vi "HOST_feedback+datatrig_AAoptAOD_9-20-23.vi"() -> ()   [LabVIEW 2020]
uses:
  <vilib>/rvi/interface/nirviMethod/nirviMethod.xnode
  <vilib>/rvi/errors/niLvFpgaMergeErrorWithErrorCode.vi
  <instrlib>/_niInstr/Streaming/v1/Host/niInstr Streaming v1 Host.lvlib
  <vilib>/rvi/interface/nirviReadWriteControl/nirviReadWriteControl.xnode
  <vilib>/rvi/interface/nirviCloseFPGA/nirviCloseFPGA.xnode
  <vilib>/rvi/interface/nirviOpenFPGA/nirviOpenFPGA.xnode
  <vilib>/rvi/interface/Simulation/niFpgaSimulationCallBeginRW.vi
  <vilib>/rvi/errors/niLvFpgaAdjustHostInterfaceError.vi
  NiFpgaLv.dll
  <vilib>/Utility/error.llb/Error Cluster From Error Code.vi
  <vilib>/Utility/file.llb/Write Delimited Spreadsheet (string).vi
  <instrlib>/_niInstr/Streaming/v1/Host/Public/Start Finite Stream.vi
  <instrlib>/_niInstr/Streaming/v1/Host/Public/Wait for Stream.vi
  <vilib>/FPGAPlugInAG/Dynamic/niLvFpga_ConfigureFifo_Dynamic.vi
  <vilib>/FPGAPlugInAG/Dynamic/niLvFpga_StartFifo_Dynamic.vi
  <vilib>/measure/NI_MAPro.lvlib
  <vilib>/measure/maspectr.llb/FFT Power Spectrum and PSD for N Chan.vi
  <instrlib>/_niInstr/Streaming/v1/Host/Public/Start Continuous Stream.vi
  <vilib>/FPGAPlugInAG/Dynamic/niLvFpga_ReadFifo_Dynamic.vi
  <vilib>/FPGAPlugInAG/Dynamic/niLvFpga_WriteFifo_Dynamic.vi
  <vilib>/FPGAPlugInAG/Dynamic/niLvFpga_Close_Dynamic.vi
  FPGA Bitfiles/rfsignalsimplifi_FPGATarget_feedbackarray+da_Q0z18vTqQOY.lvbitx
  <vilib>/FPGAPlugInAG/PXIe-7972R/niLvFpga_Open_PXIe-7972R.vi
  <vilib>/rvi/interface/common/dynamic/niFpgaDynamicAddResources.vi
  <vilib>/userdefined/Silver/nirio_resource_slv.ctl
  Controls/Clock Select.ctl
  PID/Typedef/niFpgaPID_PIDGains_FXP.ctl
  PID/Typedef/niFpgaPID_SetpointWeightings_FXP.ctl
  PID/Typedef/niFpgaPID_OutputRange_FXP.ctl
  PID/Typedef/niFpgaPID_PIDActions_FXP.ctl
panel:
  out "Boolean":bool=TRUE
  out "Stream PSD":cluster{"f0":dbl, "df":dbl, "magnitude":dbl[]}[](graph)
  out "X DC Offset Check":i16[](array[numeric])
  in  "Number of files":u16=1
  in  "RF Power normalize":bool=TRUE
  in  "Save data":bool
  in  "File base name":string="Z_3mbar_i"
  in  "Save Path Directory":path=path "D:/Lab Data/test"
  out "SUM PSD":cluster{"f0":dbl, "df":dbl, "magnitude":dbl[]}[](graph)
  out "SUM":waveform(dbl)[](graph)=[{"t0"=timestamp(0 s since 1904-01-01), "dt"=0.0002, "Y"=array[1000 elements]}, {"t0"=timestamp(0 s since 1904-01-01), "dt"=0.0002, "Y"=array[1000 elements]}, {"t0"=timestamp(0 s since 1904-01-01), "dt"=0.0002, "Y"=array[1000 elements]}, {"t0"=timestamp(0 s since 1904-01-01), "dt"=0.0002, "Y"=array[1000 elements]}]
  out "Y PSD":cluster{"f0":dbl, "df":dbl, "magnitude":dbl[]}[](graph)
  out "Y":waveform(dbl)[](graph)=[{"t0"=timestamp(0 s since 1904-01-01), "dt"=0.0002, "Y"=array[1000 elements]}, {"t0"=timestamp(0 s since 1904-01-01), "dt"=0.0002, "Y"=array[1000 elements]}, {"t0"=timestamp(0 s since 1904-01-01), "dt"=0.0002, "Y"=array[1000 elements]}, {"t0"=timestamp(0 s since 1904-01-01), "dt"=0.0002, "Y"=array[1000 elements]}]
  out "X PSD":cluster{"f0":dbl, "df":dbl, "magnitude":dbl[]}[](graph)
  out "X":waveform(dbl)[](graph)=[{"t0"=timestamp(0 s since 1904-01-01), "dt"=0.0002, "Y"=array[1000 elements]}, {"t0"=timestamp(0 s since 1904-01-01), "dt"=0.0002, "Y"=array[1000 elements]}, {"t0"=timestamp(0 s since 1904-01-01), "dt"=0.0002, "Y"=array[1000 elements]}, {"t0"=timestamp(0 s since 1904-01-01), "dt"=0.0002, "Y"=array[1000 elements]}]
  in  "Set Point Initialization":bool
  in  "Feedback scaling y":fxp<+,25,4>
  in  "Y Gains":T1[](array[typedef])
  in  "X Gains":T1[](array[typedef])
  in  "Data transfer method":bool
  in  "Downsample":u16=1
  in  "Signal Delay (us)":u16=5
  out "actions":T2
  out "error":fxp<+/-,18,11>
  out "output":fxp<+/-,20,12>
  out "error 2":fxp<+/-,18,11>
  out "error 3":fxp<+/-,18,11>
  out "output 3":fxp<+/-,20,12>
  out "actions 3":T2
  out "output 2":fxp<+/-,20,12>
  out "actions 2":T2
  in  "Z Gains":T1[](array[typedef])
  in  "setpoint weighting 3":T3={"proportional weighting (1)"=1.0, "derivative weighting (0)"=0.0}
  in  "output range 3":T4={"output high (Inf)"=2000.0, "output low (-Inf)"=-2000.0}
  in  "Z reset? (F)":bool
  in  "setpoint weighting 2":T3={"proportional weighting (1)"=1.0, "derivative weighting (0)"=0.0}
  in  "output range 2":T4={"output high (Inf)"=2000.0, "output low (-Inf)"=-2000.0}
  in  "Y reset? (F)":bool
  in  "Feedback scaling z":fxp<+,32,4>
  in  "Feedback scaling x":fxp<+,25,4>
  in  "Apply feedback":bool
  in  "Data Trigger Level (V)":dbl
  in  "Record Size":u32=1024
  out "AI":waveform(dbl)[](graph)
  in  "Data Trigger When":enum8{"Trigger Above", "Trigger Below"}(ring)
  in  "Trigger Type":enum8{"Immediate", "Data Trigger", "TRIG input"}(ring)
  in  "Direction switch":bool
  in  "Step gain values":dbl
  in  "?":bool
  in  "% of max CH 1":dbl=85.0
  in  "% of max CH 0":dbl=90.0
  in  "setpoint weighting":T3={"proportional weighting (1)"=1.0, "derivative weighting (0)"=0.0}
  in  "output range":T4={"output high (Inf)"=2000.0, "output low (-Inf)"=-2000.0}
  in  "X reset? (F)":bool
  in  "write time ch0":bool
  in  "Record time for power sweep CH0":bool
  in  "Record time for power sweep CH1":bool
  in  "write time ch1":bool
  in  "save path for power calibration (dialog if empty)":path
  out "time check":u16=16
  in  "Cycles per step":u16=30
  in  "Gain Scan Endpoint (CH1)":dbl[](array[numeric])=[100.0, 100.0, 100.0, 100.0, 100.0, 100.0, 100.0, 100.0, 100.0, 100.0, 100.0, 100.0, 100.0, 100.0, 100.0, 100.0, 100.0, 100.0, 100.0, 100.0, 100.0, 100.0, 100.0, 100.0, 100.0, 100.0, 100.0, 100.0, 100.0, 100.0, 100.0, 100.0, 100.0, 100.0, 100.0, 100.0]
  in  "Gain Scan Endpoint (CH0)":dbl[](array[numeric])=[100.0, 100.0, 100.0, 100.0, 100.0, 100.0, 100.0, 100.0, 100.0, 100.0, 100.0, 100.0, 100.0, 100.0, 100.0, 100.0, 100.0, 100.0, 100.0, 100.0, 100.0, 100.0, 100.0, 100.0, 100.0, 100.0, 100.0, 100.0, 100.0, 100.0, 100.0, 100.0, 100.0, 100.0, 100.0, 100.0]
  in  "Scan End Setpoint (CH1)":dbl[](array[numeric])=[23.0, 24.0, 25.0, 26.0, 27.0, 28.0, 23.0, 24.0, 25.0, 26.0, 27.0, 28.0, 23.0, 24.0, 25.0, 26.0, 27.0, 28.0, 23.0, 24.0, 25.0, 26.0, 27.0, 28.0, 23.0, 24.0, 25.0, 26.0, 27.0, 28.0, 23.0, 24.0, 25.0, 26.0, 27.0, 28.0] format="%#_10f"
  in  "Scan CH1":bool
  in  "Scan CH0":bool
  in  "Fq Scan Endpoint (CH0)":dbl[](array[numeric])=[23.0, 23.0, 23.0, 23.0, 23.0, 23.0, 24.0, 24.0, 24.0, 24.0, 24.0, 24.0, 25.0, 25.0, 25.0, 25.0, 25.0, 25.0, 26.0, 26.0, 26.0, 26.0, 26.0, 26.0, 27.0, 27.0, 27.0, 27.0, 27.0, 27.0, 28.0, 28.0, 28.0, 28.0, 28.0, 28.0] format="%#_10f"
  in  "Gain Scan Step Size % (CH1)":dbl=1.0
  in  "Gain Scan Step Size % (CH0)":dbl=1.0
  in  "Fq Scan Step Size MHz (CH1)":dbl=0.1
  in  "Fq Scan Step Size MHz (CH0)":dbl=0.1
  in  "Input pass through\nmode":enum16{"Wire", "Accum-edge"}(ring)=enum."Accum-edge"
  in  "# of beams":u8=36
  in  "Wave Reader CH 1 (MHz)":dbl[](array[numeric])=[23.0, 24.0, 25.0, 26.0, 27.0, 28.0, 23.0, 24.0, 25.0, 26.0, 27.0, 28.0, 23.0, 24.0, 25.0, 26.0, 27.0, 28.0, 23.0, 24.0, 25.0, 26.0, 27.0, 28.0, 23.0, 24.0, 25.0, 26.0, 27.0, 28.0, 23.0, 24.0, 25.0, 26.0, 27.0, 28.0] format="%#_15f"
  in  "Gain CH 1 (%)":dbl[](array[numeric])=[100.0, 100.0, 100.0, 100.0, 100.0, 100.0, 100.0, 100.0, 100.0, 100.0, 100.0, 100.0, 100.0, 100.0, 100.0, 100.0, 100.0, 100.0, 100.0, 100.0, 100.0, 100.0, 100.0, 100.0, 100.0, 100.0, 100.0, 100.0, 100.0, 100.0, 100.0, 100.0, 100.0, 100.0, 100.0, 100.0]
  in  "Remove transition edges":u16=5
  in  "Time per beam in us":u16=20
  in  "stop":bool
  in  "Gain CH 0 (%)":dbl[](array[numeric])=[100.0, 100.0, 100.0, 100.0, 100.0, 100.0, 100.0, 100.0, 100.0, 100.0, 100.0, 100.0, 100.0, 100.0, 100.0, 100.0, 100.0, 100.0, 100.0, 100.0, 100.0, 100.0, 100.0, 100.0, 100.0, 100.0, 100.0, 100.0, 100.0, 100.0, 100.0, 100.0, 100.0, 100.0, 100.0, 100.0]
  in  "Wave Reader CH 0 (MHz)":dbl[](array[numeric])=[23.0, 23.0, 23.0, 23.0, 23.0, 23.0, 24.0, 24.0, 24.0, 24.0, 24.0, 24.0, 25.0, 25.0, 25.0, 25.0, 25.0, 25.0, 26.0, 26.0, 26.0, 26.0, 26.0, 26.0, 27.0, 27.0, 27.0, 27.0, 27.0, 27.0, 28.0, 28.0, 28.0, 28.0, 28.0, 28.0] format="%#_13f"
  in  "Magnitude Initialization Vpp":dbl[](array[numeric])=[1.0, 1.0] format="%0.2p"
  in  "Frequencies (Hz)":dbl[](array[numeric])=[10000.0, 10000.0] format="%5.0p"
  in  "Signal Type":T5(ring)
  in  "Sampling Info":cluster{"Fs":dbl, "#s":dbl}={"Fs"=163840000.0, "#s"=32768.0} {"Fs" format="%#_5p"}
  out "Error Out":errorcluster
  in  "Update Waveform":bool
  in  "Clock Select":T6 items=["Internal Clock", "Internal Clock w/ Ref via CLK/REF IN", "Internal Clock w/ Ref via Sync Clock", "External Clock via CLK/REF IN"]
  in  "Rate of External Sample Clock (MHz)":u16=100 min=60 max=100 step=1
  in  "RIO Resource":T7="RIO0"
  # "For collecting the time and frequency when doing calibration"
  # "General Feedback Settings"
  # "Time cycle loop processing"
  # "up to 65535"
  # "Waveform Initialization"
  # "Controls the Output of the FPGA\nEach row corresponds to one beam created by the AOD\nCH 0 is Output 0 on the FPGA card and controls the () direction on the AOD; CH 1 is Output 1 on the FPGA card and controls the () direction on the AOD\n\nThe  set frequency is the output of the FPGA, this is then mixed with a 50MHz LO to be in the AOD's bandwidth of 75 +- 15MHz\n\nThe gain is the percentage of the 1Vpp initialized voltage to output. It is in percentage and goes from 0 - 100\n\nIt will play the first n rows of tones, \nwhere n is the \"# of beams\" value."
  # "DO NOT CHANGE"
  # "These allow you to smoothly ramp between frequencies or gain settings for each individual beam.\nThe channels scan independently, but it will simultaneously ramp every fq/gain in the channel to their desired point.\nThey should update to match the main control setting when scanning is not enabled."
  # "X Feedback"
  # "Do not change these values while waiting for scan"
  # "Main control for the tones played on FPGA analog out 0\nSets the base, static frequency to play"
  # "Main control for the tones played on FPGA analog out 1\nSets the base, static frequency to play"
  # "Don't change"
  # "Ch 0 Output Waveforms"
  # "Ch 1 Output Waveforms"
  # "Y Feedback"
  # "Ch0"
  # "Ch1"
  # "Makes sure the RF power into the\nAOD is flattened to 1.7W across the\nbandwidth\nDO NOT TURN OFF UNLESS YOU\nARE CALIBRATING POWERS!\nWILL BREAK THE AOD!"
  # "Z Feedback"
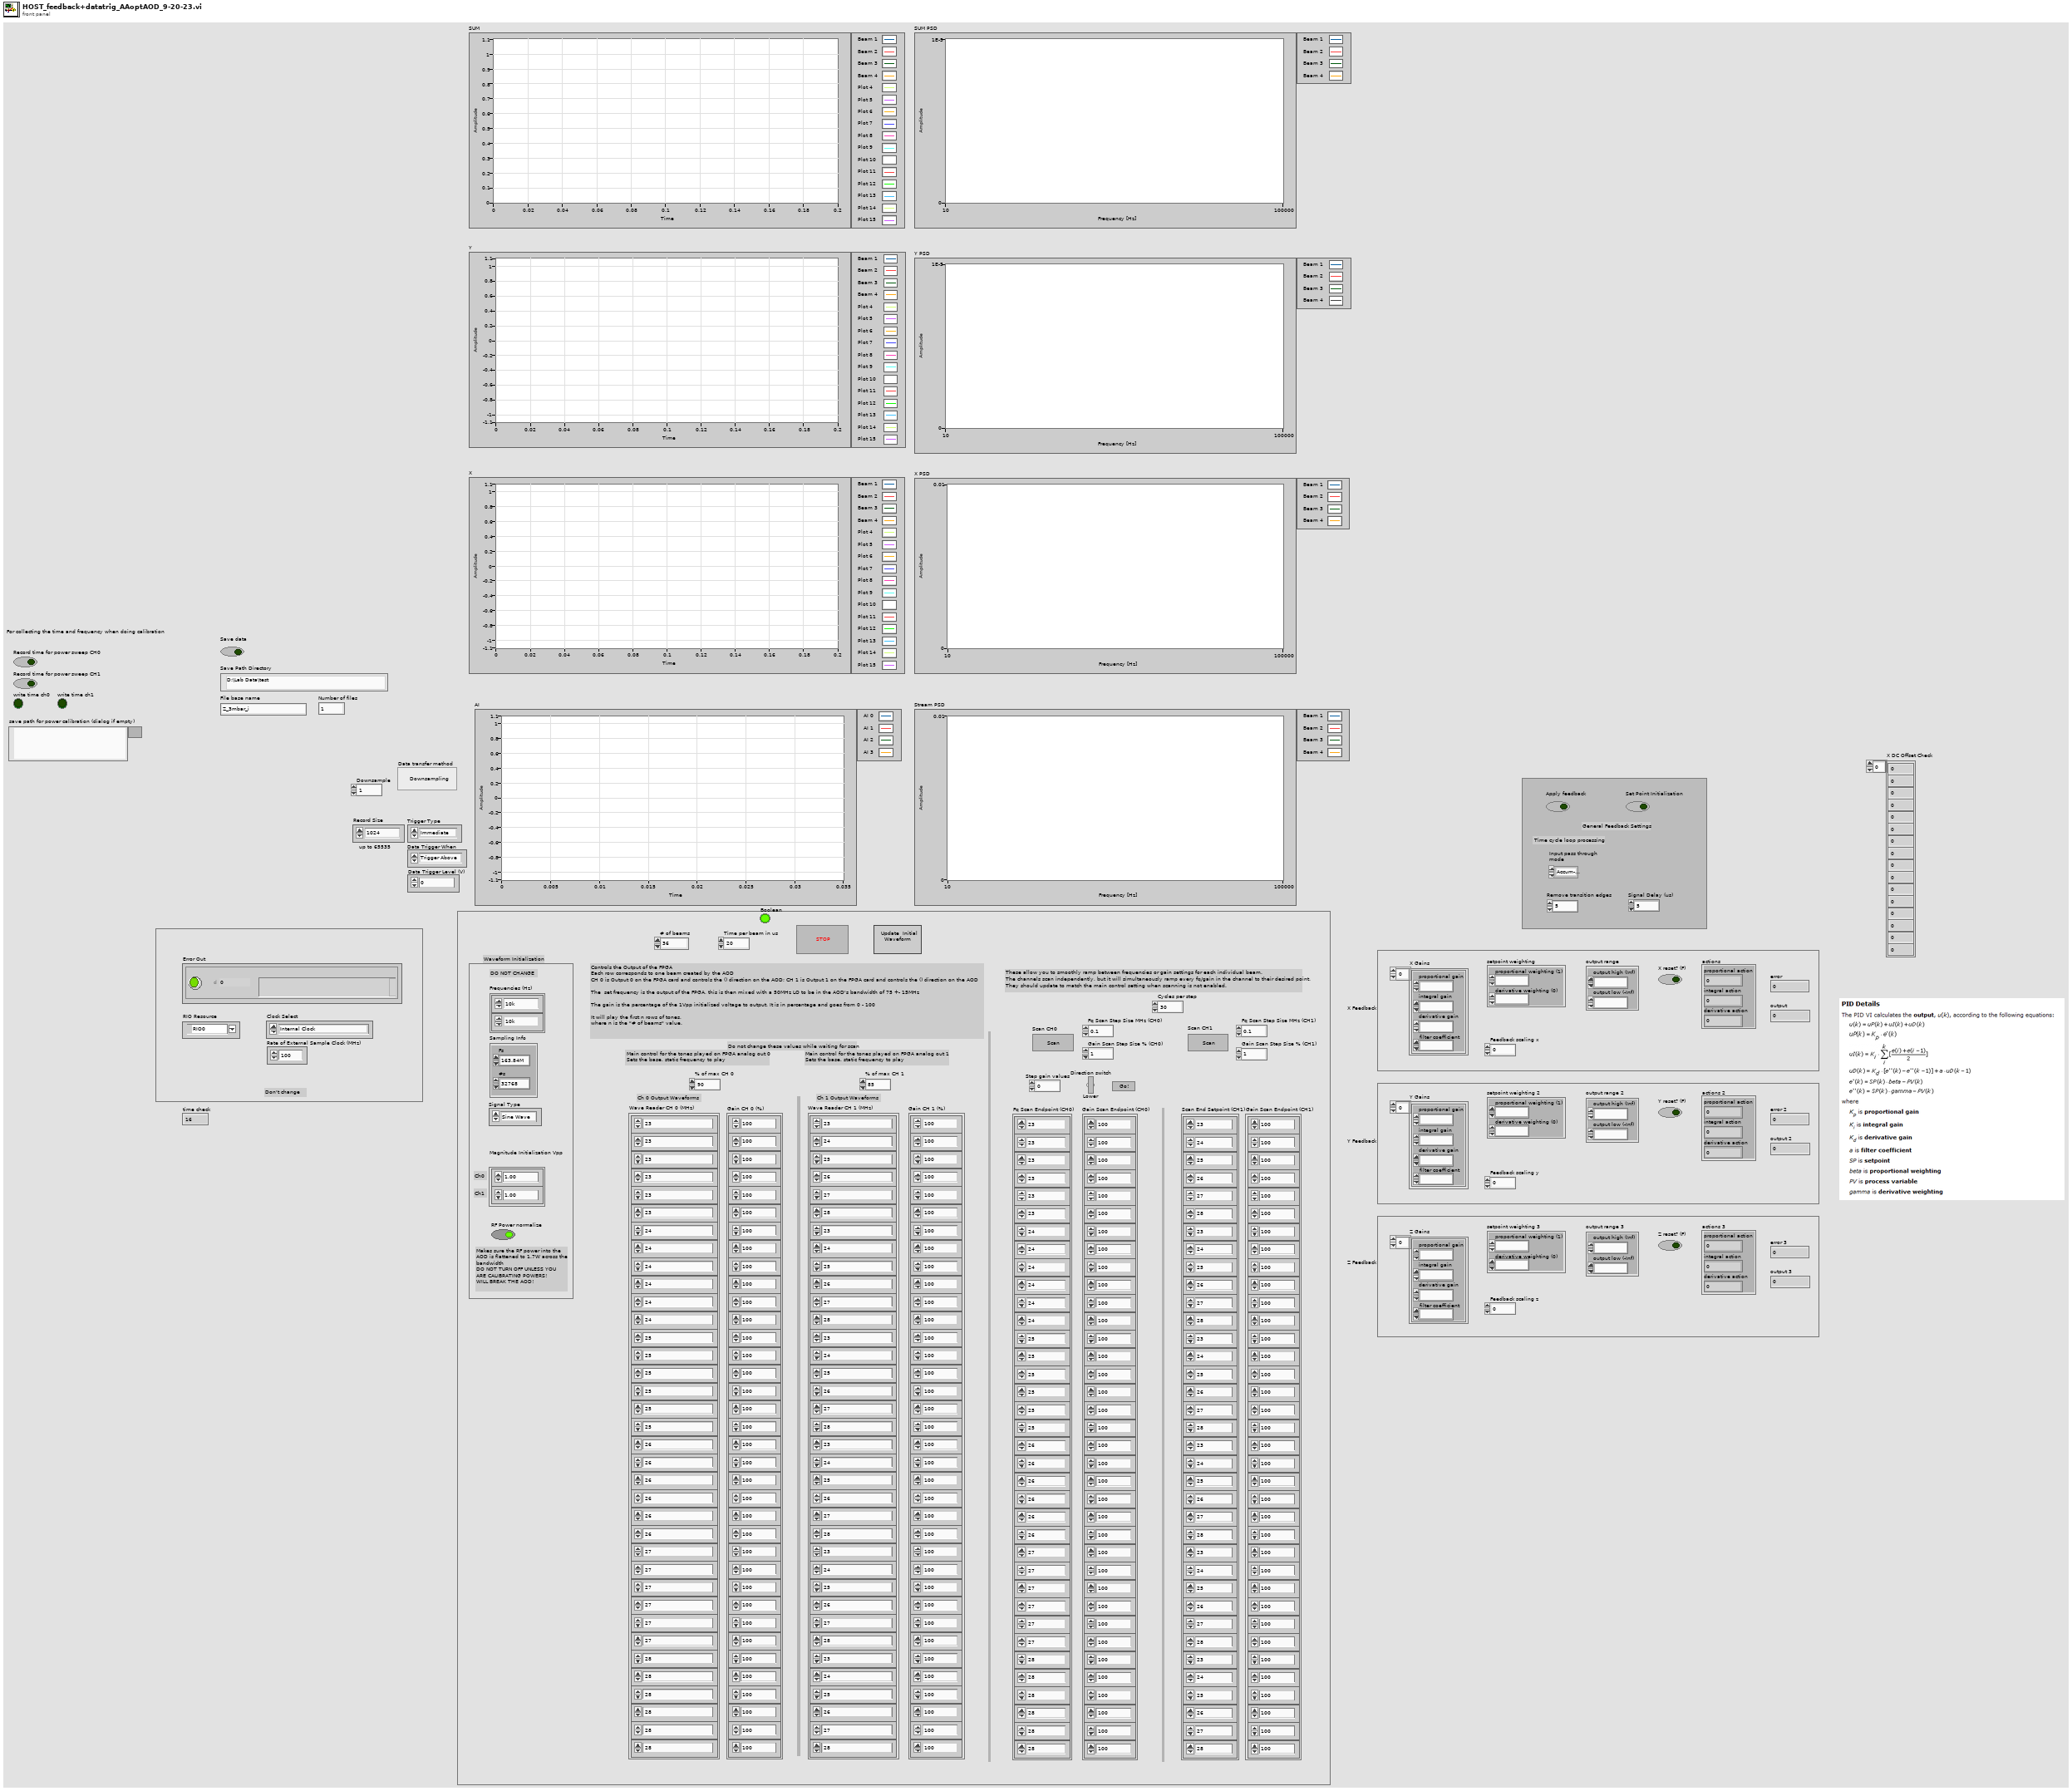
[diagram p1: front panel]
types:
  T1 = typedef "niFpgaPID_PIDGains_FXP.ctl" = cluster{"proportional gain":fxp<+/-,17,4>, "integral gain":fxp<+/-,16,3>, "derivative gain":fxp<+/-,16,3>, "filter coefficient":fxp<+/-,17,4>}
  T2 = typedef "niFpgaPID_PIDActions_FXP.ctl" = cluster{"proportional action":fxp<+/-,20,12>, "integral action":fxp<+/-,20,12>, "derivative action":fxp<+/-,20,12>}
  T3 = typedef "niFpgaPID_SetpointWeightings_FXP.ctl" = cluster{"proportional weighting (1)":fxp<+/-,16,2>, "derivative weighting (0)":fxp<+/-,16,2>}
  T4 = typedef "niFpgaPID_OutputRange_FXP.ctl" = cluster{"output high (Inf)":fxp<+/-,20,12>, "output low (-Inf)":fxp<+/-,20,12>}
  T5 = enum16{"Sine Wave", "Triangle Wave", "Square Wave", "Sawtooth Wave"}
  T6 = typedef "Clock Select.ctl" = u16
  T7 = typedef "nirio_resource_slv.ctl" = tag
  T8 = cluster{"level":i16, "trigger when":enum8{"Trigger Above", "Trigger Below"}}
  T9 = cluster{"proportional action":sgl, "integral action":sgl, "derivative action":sgl}
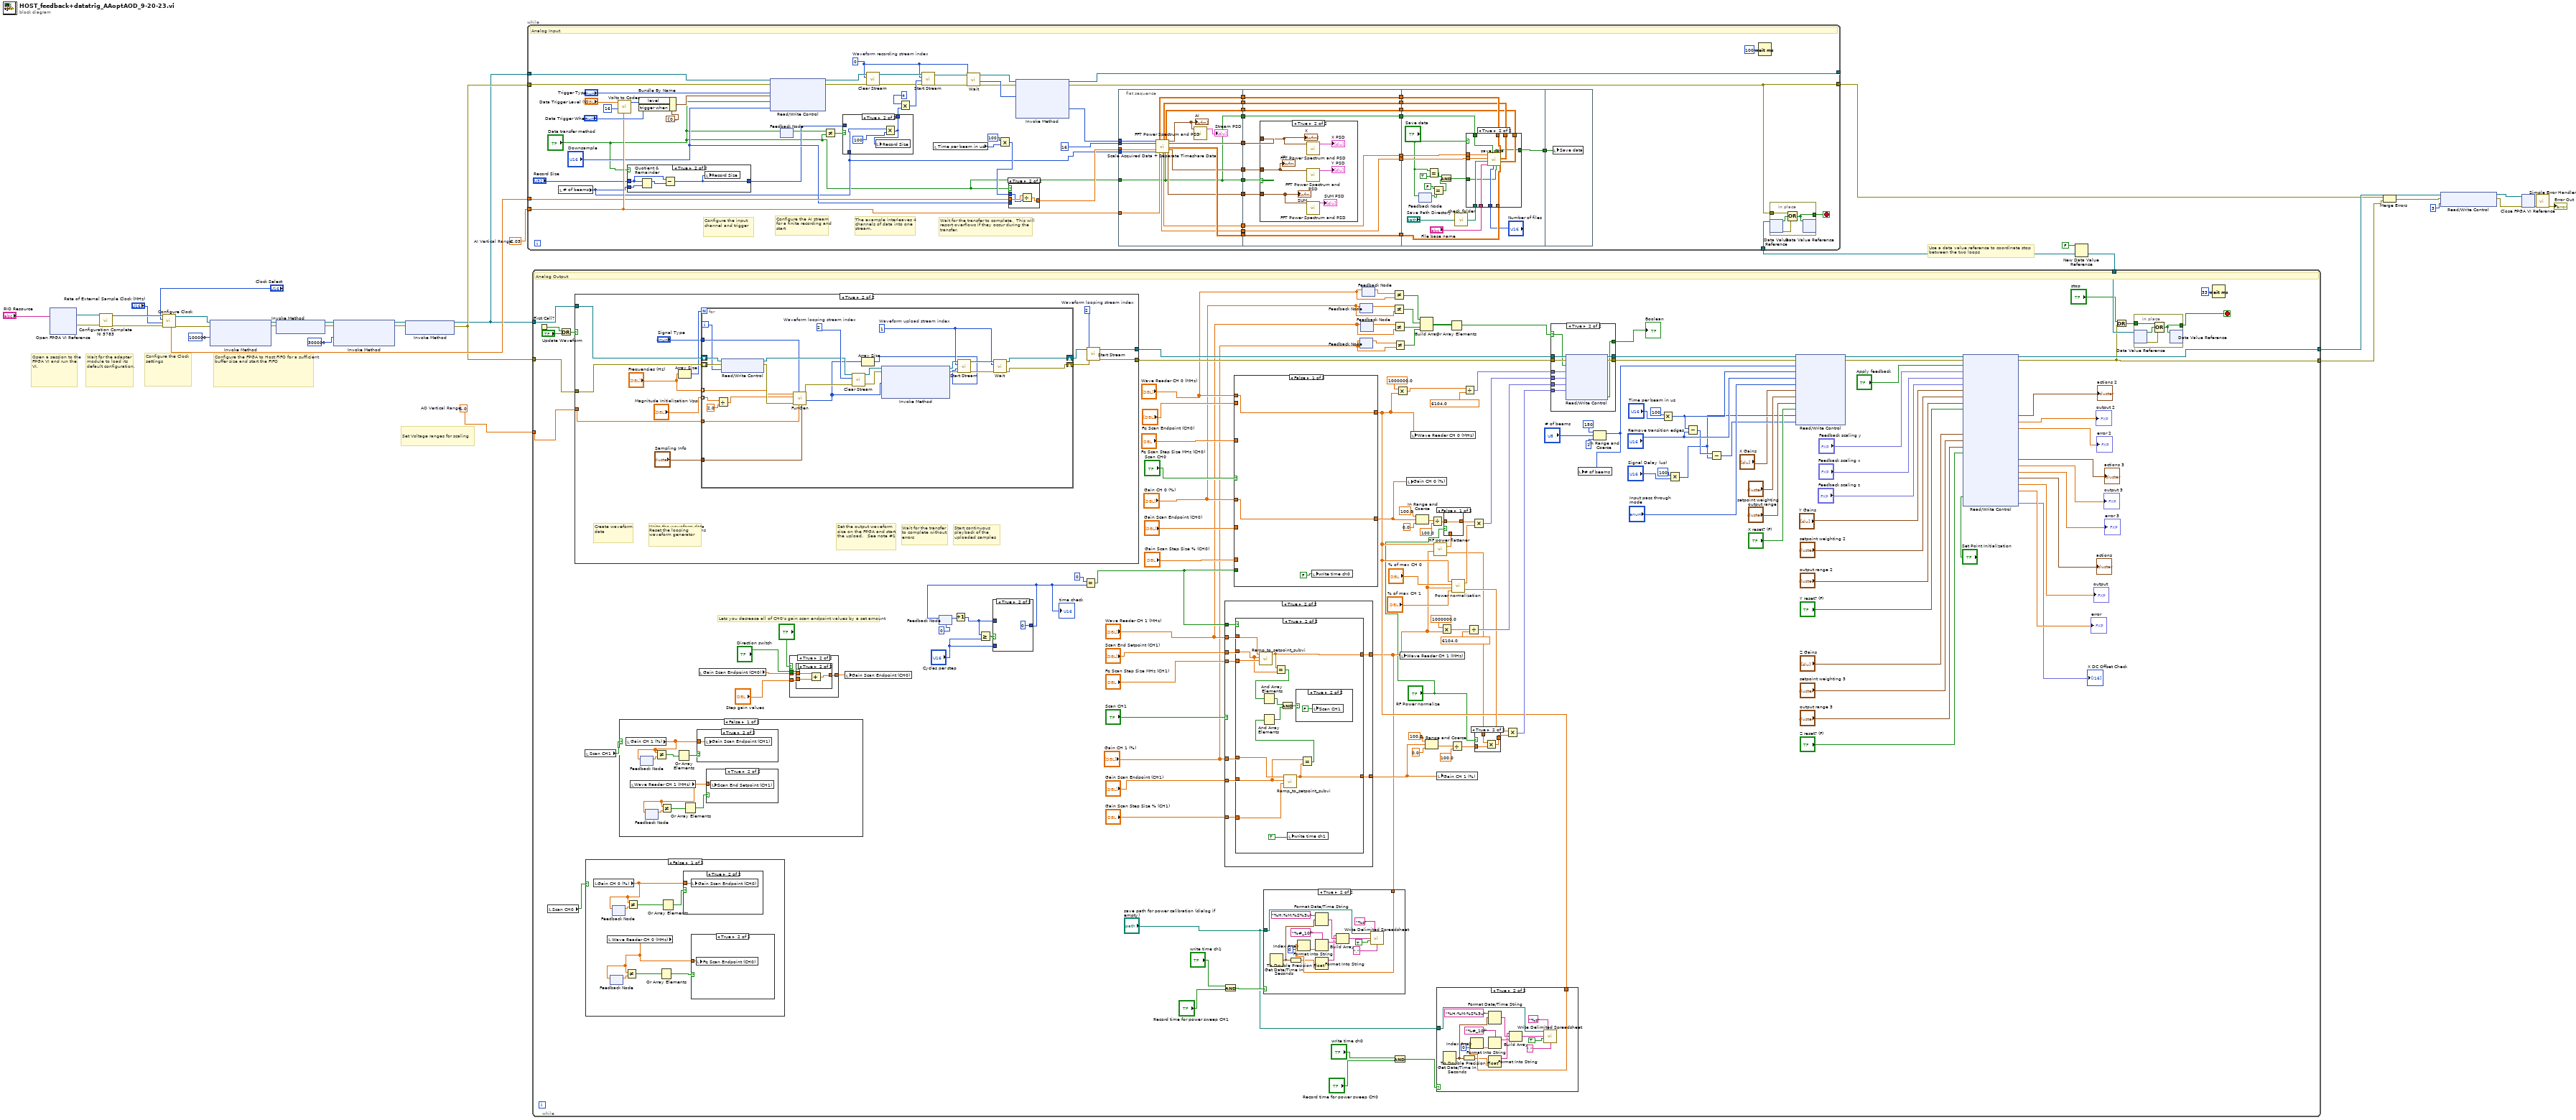
[diagram p0: block diagram]
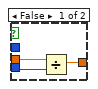
[diagram p6: hidden frame]
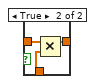
[diagram p8: hidden frame]
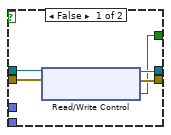
[diagram p9: hidden frame]
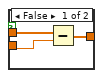
[diagram p11: hidden frame]
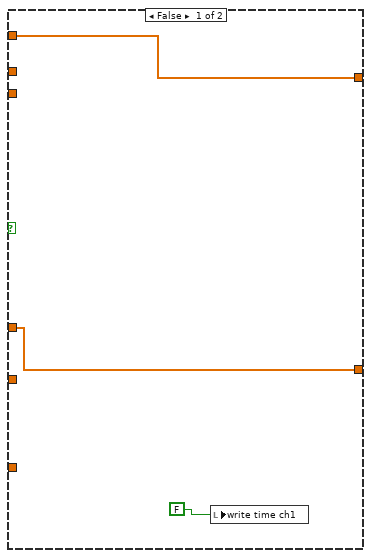
[diagram p14: hidden frame]
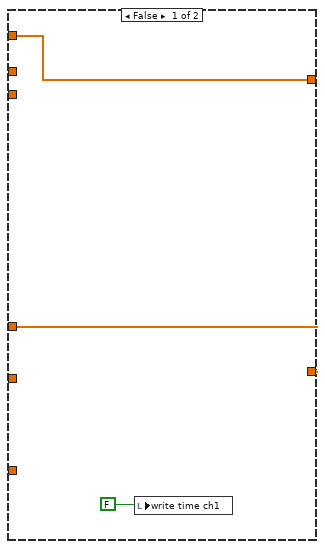
[diagram p15: hidden frame]
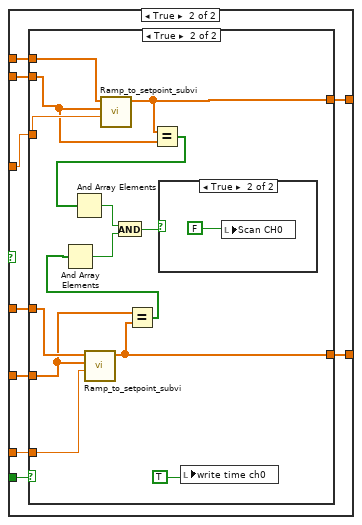
[diagram p17: hidden frame]
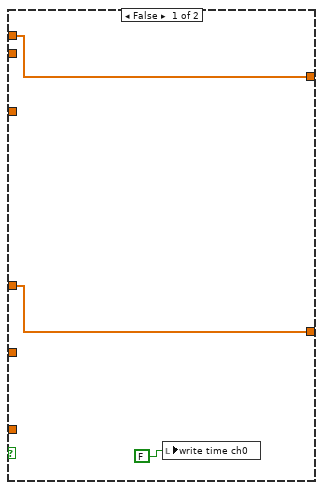
[diagram p18: hidden frame]
diagram:
  w13 = 2.03  # AI Vertical Range
  w21 = 1.0  # AO Vertical Range
  # "Use a data value reference to coordinate stop between the two loops"
  # "Set Voltage ranges for scaling"
  # "Configure the Clock settings"
  # "Configure the FPGA to Host FIFO for a sufficient buffer size and start the FIFO"
  # "Wait for the adapter module to load its default configuration."
  # "Open a session to the FPGA VI and run the VI."
  n1 = xnode "Open FPGA VI Reference"("resource name"="RIO Resource") -> ("FPGA VI Reference Out"=w19:refnum<k20>, "error out"=w18:errorcluster)  [unwired: 1 in]
  n2 = call "Configuration Complete NI 5783.vi"("error in"=w18, "FPGA VI Reference In"=w19) -> ("error out"=w29:errorcluster, "FPGA VI Reference Out"=w30:refnum<k20>)  [unwired: 7 in, 1 out]
  n3 = call "Configure Clock.vi"("error in (no error)"=w29, "Rate of External Sample Clock (MHz)"="Rate of External Sample Clock (MHz)", "Clock Select"="Clock Select", "FPGA VI Reference In"=w30) -> ("error out"=w27:errorcluster, "FPGA VI Reference Out"=w28:refnum<k20>, "Sampling Rate"=w12:dbl)  [unwired: 3 in, 2 out]
  n4 = xnode "Invoke Method"("FPGA VI Reference In"=w28, "error in"=w27, "Requested Depth"=u32 100000) -> ("FPGA VI Reference Out"=w33:refnum<k20>, "error out"=w32:errorcluster)  [unwired: 1 out]
  n5 = xnode "Invoke Method"("FPGA VI Reference In"=w33, "error in"=w32) -> ("FPGA VI Reference Out"=w5:refnum<k20>, "error out"=w8:errorcluster)
  n6 = xnode "Invoke Method"("FPGA VI Reference In"=w5, "error in"=w8, "Requested Depth"=u32 300000) -> ("FPGA VI Reference Out"=w4:refnum<k20>, "error out"=w7:errorcluster)  [unwired: 1 out]
  n7 = xnode "Invoke Method"("FPGA VI Reference In"=w4, "error in"=w7) -> ("FPGA VI Reference Out"=w3:refnum<k20>, "error out"=w6:errorcluster)
  n8 = New Data Value Reference(data value=FALSE ("Stopped")) -> (data value reference=w1:refnum<data-value>)  [unwired: 1 in, 1 out]
  n9 = while {
    tunnel: [w93] -> _
    tunnel: w3 -> [w92]
    tunnel: w13 -> [w76]
    tunnel: w1 -> [w89]
    tunnel: w6 -> [w91]
    tunnel: [w80] -> w10
    tunnel: w12 -> [w67]
    stop <- w90 stop-if-true
    w70 = 0  # Waveform recording stream index
    # "The example interleaves 4 channels of data into one stream."
    # "Wait for the transfer to complete.  This will report overflows if they occur during the transfer."
    # "Configure the AI stream for a finite recording and start"
    # "Configure the input channel and trigger"
    # "Analog Input"
    n10 = local read "# of beams"() -> (w55:u8)
    n11 = call "Volts to Codes.vi"("range (Vpp)"=w76, "Number of Bits"=i16 16, "Volts In"="Data Trigger Level (V)") -> ("ADC Codes Out"=w77:i16)  [unwired: 8 in]
    n12 = case shown="True" "Data transfer method" {
      tunnel: "Record Size" -> [w162 w165]
      tunnel: [w162 w163] -> w59
      tunnel: w55 -> [_ w166]
      frame False {
      }
      frame True {
        n13 = Quotient & Remainder(x=w165, y=w166) -> (x-y*floor(x/y)=w164:u32)  [unwired: 1 out]
        n14 = Subtract(x=w165, y=w164) -> (x-y=w163:u32)
        n15 = local write "Record Size"(w163) -> ()
      }
    }
    n16 = Bundle By Name(cluster=T8 {"level"=0, "trigger when"=enum."Trigger Above"} ("Trigger Configuration"), "level"=w77, "trigger when"="Data Trigger When") -> (w69:T8)
    n17 = xnode "Read/Write Control"("FPGA VI Reference In"=w92, "error in"=w91, "Trigger Type"="Trigger Type", "Trigger Configuration"=w69, "Data transfer method"="Data transfer method", "Downsample"="Downsample") -> ("FPGA VI Reference Out"=w74:refnum<k20>, "error out"=w73:errorcluster)
    n18 = feedback-in #1("Data transfer method") -> ()
    n19 = feedback #1() -> (w60:bool)  [unwired: 1 in]
    n20 = Not Equal?(x=w60, y="Data transfer method") -> (x != y?=w61:bool)
    n21 = case shown="True" w61 {
      tunnel: w59 -> [w167 _]
      tunnel: [w167 w170] -> w58
      tunnel: w55 -> [_ w168]
      frame False {
      }
      frame True {
        n22 = Multiply(x=w168, y=100) -> (x*y=w170:u32)
        n23 = local write "Record Size"(w170) -> ()
      }
    }
    n24 = call <instrlib>:"Clear Stream.vi"("error in (no error)"=w73, "stream index"=w70, "refnum in"=w74) -> ("error out"=w72:errorcluster, "refnum out"=w71:refnum<k20>)  [unwired: 7 in]
    n25 = Multiply(x=u16 4 ("y"), y=w58) -> (x*y=w75:u32)
    n26 = call-poly <instrlib>:"Start Stream.vi"("error in (no error)"=w72, "num samples"=w75, "stream index"=w70, "refnum in"=w71) -> ("error out"=w85:errorcluster, "refnum out"=w83:refnum<k20>)  [unwired: 6 in]
    n27 = local read "Time per beam in us"() -> (w63:u16)
    n28 = call-poly <instrlib>:"Wait.vi"("error in (no error)"=w85, "stream index"=w70, "refnum in"=w83) -> ("error out"=w81:errorcluster, "samples transferred"=w84:u64, "refnum out"=w82:refnum<k20>)  [unwired: 5 in, 1 out]
    n29 = Multiply(x=100, y=w63) -> (x*y=w56:i32)
    n30 = case shown="True" "Data transfer method" {
      tunnel: w67 -> [w173 w176]
      tunnel: [w172 w174] -> w66
      tunnel: "Downsample" -> [w171 _]
      tunnel: w56 -> [_ w175]
      frame False {
        n31 = Divide(x=w173, y=w171) -> (x/y=w172:dbl)
      }
      frame True {
        n32 = Divide(x=w176, y=w175) -> (x/y=w174:dbl)
      }
    }
    n33 = xnode "Invoke Method"("FPGA VI Reference In"=w82, "error in"=w81, "Number of Elements"=w84) -> ("FPGA VI Reference Out"=w93:refnum<k20>, "error out"=w80:errorcluster, "Data"=w62:i16[])  [unwired: 1 in, 1 out]
    n34 = flat-sequence {
      tunnel: i16 16 ("Number of Bits") -> [w111]
      tunnel: w76 -> [w110]
      tunnel: w66 -> [w109]
      tunnel: w62 -> [w108]
      tunnel: w55 -> [w101]
      tunnel: "Data transfer method" -> [w97]
      tunnel: [w107] -> w52
      tunnel: [w106] -> w50
      tunnel: [w105] -> w48
      tunnel: [w104] -> w46
      tunnel: [w103] -> w44
      tunnel: [w102] -> w42
      tunnel: [w97] -> w40
      tunnel: [w100] -> w37
      tunnel: [w99] -> w36
      tunnel: [w98] -> w35
      tunnel: [w97] -> w34
      tunnel: w52 -> [w122]
      tunnel: [w122] -> w51
      tunnel: w50 -> [w121]
      tunnel: [w121] -> w49
      tunnel: w48 -> [w120]
      tunnel: [w120] -> w47
      tunnel: w46 -> [w119]
      tunnel: [w119] -> w45
      tunnel: w44 -> [w118]
      tunnel: [w118] -> w43
      tunnel: w42 -> [w117]
      tunnel: [w117] -> w41
      tunnel: w40 -> [w116]
      tunnel: [w116] -> w39
      tunnel: w37 -> [w115]
      tunnel: w36 -> [w114]
      tunnel: w35 -> [w113]
      tunnel: w34 -> [w112]
      tunnel: w51 -> [w144]
      tunnel: w49 -> [w143]
      tunnel: w47 -> [w142]
      tunnel: w45 -> [w141]
      tunnel: w43 -> [w137]
      tunnel: w41 -> [w138]
      tunnel: w39 -> [w139]
      tunnel: [w140] -> w53
      tunnel: w53 -> [w161]
      frame #0 {
        n35 = call "Scale Acquired Data + Separate Timeshare Data.vi"("Data In"=w108, "Number of Bits"=w111, "Sample Rate"=w109, "Array size"=w101, "range (V)"=w110, "Timeshare sampling"=w97) -> ("Beam sorted X data"=w107:dbl[][], "AI stream sampling rate"=w102:dbl, "Beam sorted Y data"=w106:dbl[][], "Beam sorted sampling rate"=w103:dbl, "Beam sorted SUM data"=w105:dbl[][], "Data"=w95:waveform(dbl)[], "X Data"=w100:waveform(dbl)[], "AI stream data"=w104:dbl[][], "Y Data"=w99:waveform(dbl)[], "SUM Data"=w98:waveform(dbl)[])  [unwired: 4 in]
        "AI" <- w95
        n36 = call-poly <vilib>:"FFT Power Spectrum and PSD.vi"("time signals"=w95) -> ("Power Spectrum / PSD"=→"Stream PSD":cluster{"f0":dbl, "df":dbl, "magnitude":dbl[]}[])  [unwired: 7 in, 3 out]
      }
      frame #1 {
        n37 = case shown="True" w112 {
          tunnel: w115 -> [_ w128]
          tunnel: w114 -> [_ w124]
          tunnel: w113 -> [_ w123]
          frame False {
          }
          frame True {
            n38 = call-poly <vilib>:"FFT Power Spectrum and PSD.vi"("time signals"=w128) -> ("Power Spectrum / PSD"=→"X PSD":cluster{"f0":dbl, "df":dbl, "magnitude":dbl[]}[])  [unwired: 7 in, 3 out]
            n39 = call-poly <vilib>:"FFT Power Spectrum and PSD.vi"("time signals"=w124) -> ("Power Spectrum / PSD"=→"Y PSD":cluster{"f0":dbl, "df":dbl, "magnitude":dbl[]}[])  [unwired: 7 in, 3 out]
            n40 = call-poly <vilib>:"FFT Power Spectrum and PSD.vi"("time signals"=w123) -> ("Power Spectrum / PSD"=→"SUM PSD":cluster{"f0":dbl, "df":dbl, "magnitude":dbl[]}[])  [unwired: 7 in, 3 out]
            "X" <- w128
            "Y" <- w124
            "SUM" <- w123
          }
        }
      }
      frame #2 {
        n41 = feedback-in #2("Save data") -> ()
        n42 = feedback #2() -> (w136:bool)  [unwired: 1 in]
        n43 = Equal?(x="Save data", y=TRUE) -> (x = y?=w132:bool)
        n44 = Equal?(x=FALSE, y=w136) -> (x = y?=w131:bool)
        n45 = And(x=w132, y=w131) -> (x .and. y?=w129:bool)
        n46 = call "check_folder.vi"("path in"="Save Path Directory") -> ("path out"=w146:path)
        n47 = case shown="True" "Save data" {
          selector: "Save data" -> [w148 _]
          tunnel: w146 -> [_ w160]
          tunnel: "File base name" -> [_ w159]
          tunnel: w144 -> [_ w158]
          tunnel: w143 -> [_ w157]
          tunnel: w142 -> [_ w156]
          tunnel: w141 -> [_ w155]
          tunnel: w137 -> [_ w154]
          tunnel: w138 -> [_ w153]
          tunnel: [w148 w152] -> w140
          tunnel: w139 -> [_ w151]
          tunnel: "Number of files" -> [_ w150]
          tunnel: w129 -> [_ w149]
          frame False {
          }
          frame True {
            n48 = call "save_data.vi"("AI stream data"=w155, "Beam sorted SUM data"=w156, "Beam sorted Y data"=w157, "Beam sorted X data"=w158, "Reset file counter"=w149, "Number of files"=w150, "Collection type"=w151, "File name"=w159, "Save Path Directory"=w160, "AI stream sampling rate"=w153, "Beam sorted sampling rate"=w154) -> ("Saving"=w152:bool)
          }
        }
      }
      frame #3 {
        n49 = local write "Save data"(w161) -> ()
      }
    }
    n50 = Wait (ms)(milliseconds to wait=u32 100) -> ()  [unwired: 1 out]
    n51 = in-place {
      in-place-border: [w178] -> w90
      in-place-border: w80 -> [w180]
      n52 = in-place-dvr #3(w89) -> (w179:bool, w177:errorcluster)
      n53 = Compound Arithmetic op=OR(w180, w179, w177) -> (w178:bool)
      n54 = in-place-dvr #3(w178) -> ()  [unwired: 2 out]
    }
  }
  n55 = while {
    tunnel: w6 -> [w314]
    tunnel: w3 -> [w320]
    tunnel: [w240] -> w17
    tunnel: w1 -> [w315]
    tunnel: w21 -> [w313]
    tunnel: [w238] -> w9
    stop <- w245 stop-if-true
    # "Lets you decrease all of CH0's gain scan endpoint values by a set amount"
    # "Analog Output"
    n56 = First Call?() -> (First Call?: T/F=w316:bool)
    n57 = local read "Scan CH0"() -> (w283:bool)
    n58 = Or(x=w316, y="Update Waveform") -> (x .or. y?=w317:bool)
    n59 = case shown="True" w317 {
      tunnel: [w472 w485] -> w312
      tunnel: [w471 w484] -> w311
      tunnel: w320 -> [w472 w482]
      tunnel: w314 -> [w471 w481]
      tunnel: w313 -> [_ w483]
      frame False {
      }
      frame True {
        w480 = 2  # Waveform looping stream index
        # "Loop over the waveforms to combine"
        # "Reset the looping waveform generator"
        # "Start continuous playback of the uploaded samples"
        # "Wait for the transfer to complete without errors"
        # "Set the output waveform size on the FPGA and start the upload.   See note #1"
        # "Write the waveform data to the FPGA for generation"
        # "Create waveform data"
        n60 = Array Size(array="Frequencies (Hz)") -> (size(s)=w475:i32)
        n61 = for {
          N: w475 -> [_]
          tunnel: w483 -> [w500]
          shift-right: [w494] -> w479
          shift-left: w482 -> [w499]
          shift-right: [w493] -> w478
          shift-left: w481 -> [w497]
          tunnel: "Frequencies (Hz)" -> [w492] mode=indexing
          tunnel: "Magnitude Initialization Vpp" -> [w488] mode=indexing
          tunnel: "Sampling Info" -> [w491]
          tunnel: "Signal Type" -> [w490]
          i -> [w489]
          w501 = 2  # Waveform looping stream index
          w506 = 1  # Waveform upload stream index
          n62 = Divide(x=w488, y=2.0) -> (x/y=w487:dbl)
          n63 = xnode "Read/Write Control"("FPGA VI Reference In"=w499, "error in"=w497, "Upload selector"=w489) -> ("FPGA VI Reference Out"=w498:refnum<k20>, "error out"=w496:errorcluster)
          n64 = call "FunGen.vi"("sampling info"=w491, "range (Vpp)"=w500, "signal type"=w490, "error in (no error)"=w496, "amplitude"=w487, "frequency"=w492) -> ("error out"=w502:errorcluster, "Waveform Data"=w495:i16[])  [unwired: 2 in, 2 out]
          n65 = call <instrlib>:"Clear Stream.vi"("error in (no error)"=w502, "stream index"=w501, "refnum in"=w498) -> ("error out"=w504:errorcluster, "refnum out"=w505:refnum<k20>)  [unwired: 7 in]
          n66 = Array Size(array=w495) -> (size(s)=w503:i32)
          n67 = xnode "Invoke Method"("FPGA VI Reference In"=w505, "error in"=w504, "Data"=w495) -> ("FPGA VI Reference Out"=w510:refnum<k20>, "error out"=w509:errorcluster)  [unwired: 1 in, 1 out]
          n68 = call-poly <instrlib>:"Start Stream.vi"("error in (no error)"=w509, "num samples"=w503, "stream index"=w506, "refnum in"=w510) -> ("error out"=w507:errorcluster, "refnum out"=w508:refnum<k20>)  [unwired: 6 in]
          n69 = call-poly <instrlib>:"Wait.vi"("error in (no error)"=w507, "stream index"=w506, "refnum in"=w508) -> ("error out"=w493:errorcluster, "refnum out"=w494:refnum<k20>)  [unwired: 5 in, 2 out]
        }
        n70 = call-poly <instrlib>:"Start Stream.vi"("error in (no error)"=w478, "stream index"=w480, "refnum in"=w479) -> ("error out"=w484:errorcluster, "refnum out"=w485:refnum<k20>)  [unwired: 7 in]
      }
    }
    n71 = local read "Scan CH1"() -> (w284:bool)
    n72 = case shown="False" w283 {
      frame False {
        n73 = local read "Gain CH 0 (%)"() -> (w447:dbl[])
        n74 = local read "Wave Reader CH 0 (MHz)"() -> (w454:dbl[])
        n75 = feedback-in #4(w454) -> ()
        n76 = feedback #4() -> (w453:dbl[])  [unwired: 1 in]
        n77 = feedback #5() -> (w450:dbl[])  [unwired: 1 in]
        n78 = feedback-in #5(w447) -> ()
        n79 = Not Equal?(x=w454, y=w453) -> (x != y?=w452:bool[])
        n80 = Not Equal?(x=w447, y=w450) -> (x != y?=w449:bool[])
        n81 = Or Array Elements(Boolean array=w452) -> (logical OR=w451:bool)
        n82 = Or Array Elements(Boolean array=w449) -> (logical OR=w448:bool)
        n83 = case shown="True" w448 {
          tunnel: w447 -> [_ w455]
          frame False {
          }
          frame True {
            n84 = local write "Gain Scan Endpoint (CH0)"(w455) -> ()
          }
        }
        n85 = case shown="True" w451 {
          tunnel: w454 -> [_ w456]
          frame False {
          }
          frame True {
            n86 = local write "Fq Scan Endpoint (CH0)"(w456) -> ()
          }
        }
      }
      frame True {
      }
    }
    n87 = case shown="False" w284 {
      frame False {
        n88 = local read "Gain CH 1 (%)"() -> (w457:dbl[])
        n89 = local read "Wave Reader CH 1 (MHz)"() -> (w461:dbl[])
        n90 = feedback #6() -> (w460:dbl[])  [unwired: 1 in]
        n91 = feedback-in #6(w457) -> ()
        n92 = feedback #7() -> (w464:dbl[])  [unwired: 1 in]
        n93 = feedback-in #7(w461) -> ()
        n94 = Not Equal?(x=w457, y=w460) -> (x != y?=w459:bool[])
        n95 = Not Equal?(x=w461, y=w464) -> (x != y?=w463:bool[])
        n96 = Or Array Elements(Boolean array=w459) -> (logical OR=w458:bool)
        n97 = Or Array Elements(Boolean array=w463) -> (logical OR=w462:bool)
        n98 = case shown="True" w458 {
          tunnel: w457 -> [_ w465]
          frame False {
          }
          frame True {
            n99 = local write "Gain Scan Endpoint (CH1)"(w465) -> ()
          }
        }
        n100 = case shown="True" w462 {
          tunnel: w461 -> [_ w466]
          frame False {
          }
          frame True {
            n101 = local write "Scan End Setpoint (CH1)"(w466) -> ()
          }
        }
      }
      frame True {
      }
    }
    n102 = local read "Gain Scan Endpoint (CH0)"() -> (w247:dbl[])
    n103 = case shown="True" "?" {
      tunnel: w247 -> [w344 w347]
      tunnel: [w344 w348] -> w248
      tunnel: "Step gain values" -> [_ w346]
      tunnel: "Direction switch" -> [_ w345]
      frame False {
      }
      frame True {
        n104 = case shown="True" w345 {
          tunnel: [w351 w353] -> w348
          tunnel: w347 -> [w350 w352]
          tunnel: w346 -> [w349 w354]
          frame False {
            n105 = Subtract(x=w350, y=w349) -> (x-y=w351:dbl[])
          }
          frame True {
            n106 = Add(x=w352, y=w354) -> (x+y=w353:dbl[])
          }
        }
      }
    }
    n107 = local write "Gain Scan Endpoint (CH0)"(w248) -> ()
    n108 = feedback #8(u16 0) -> (w279:u16)
    n109 = Increment(x=w279) -> (x+1=w277:u16)
    n110 = Greater Or Equal?(x=w277, y="Cycles per step") -> (x >= y?=w278:bool)
    n111 = case shown="True" w278 {
      tunnel: w277 -> [w445 _]
      tunnel: "Cycles per step" -> [_ _]
      tunnel: [w445 u16 0] -> w272
      frame False {
      }
      frame True {
      }
    }
    "time check" <- w272
    n112 = feedback-in #8(w272) -> ()
    n113 = Equal?(x=u16 0, y=w272) -> (x = y?=w273:bool)
    n114 = And(x="write time ch1", y="Record time for power sweep CH1") -> (x .and. y?=w271:bool)
    n115 = case shown="True" "Scan CH1" {
      tunnel: "Fq Scan Step Size MHz (CH1)" -> [_ w396]
      tunnel: [w387 w395] -> w205
      tunnel: "Wave Reader CH 1 (MHz)" -> [w387 w394]
      tunnel: "Scan End Setpoint (CH1)" -> [_ w393]
      tunnel: "Gain Scan Step Size % (CH1)" -> [_ w392]
      tunnel: "Gain CH 1 (%)" -> [w386 w391]
      tunnel: "Gain Scan Endpoint (CH1)" -> [_ w390]
      tunnel: [w386 w389] -> w285
      tunnel: w273 -> [_ w388]
      frame False {
        n116 = local write "write time ch1"(FALSE) -> ()
      }
      frame True {
        n117 = case shown="True" w388 {
          tunnel: w394 -> [w399 w413]
          tunnel: w393 -> [_ w411]
          tunnel: w396 -> [_ w412]
          tunnel: [w399 w410] -> w395
          tunnel: w391 -> [w398 w408]
          tunnel: w390 -> [_ w407]
          tunnel: w392 -> [_ w406]
          tunnel: [w398 w401] -> w389
          frame False {
            n118 = local write "write time ch1"(FALSE) -> ()
          }
          frame True {
            n119 = call "Ramp_to_setpoint_subvi.vi"("Numeric"=w412, "Scan to Fq (CH0)"=w411, "Wave Reader CH 0 (Y)"=w413) -> ("Array"=w410:dbl[])  [unwired: 8 in]
            n120 = Equal?(x=w410, y=w411) -> (x = y?=w409:bool[])
            n121 = And Array Elements(Boolean array=w409) -> (logical AND=w403:bool)
            n122 = call "Ramp_to_setpoint_subvi.vi"("Numeric"=w406, "Scan to Fq (CH0)"=w407, "Wave Reader CH 0 (Y)"=w408) -> ("Array"=w401:dbl[])  [unwired: 8 in]
            n123 = local write "write time ch1"(TRUE) -> ()
            n124 = Equal?(x=w407, y=w401) -> (x = y?=w402:bool[])
            n125 = And Array Elements(Boolean array=w402) -> (logical AND=w404:bool)
            n126 = And(x=w403, y=w404) -> (x .and. y?=w405:bool)
            n127 = case shown="True" w405 {
              frame False {
              }
              frame True {
                n128 = local write "Scan CH1"(FALSE) -> ()
              }
            }
          }
        }
      }
    }
    n129 = case shown="False" "Scan CH0" {
      tunnel: "Fq Scan Step Size MHz (CH0)" -> [_ w426]
      tunnel: "Wave Reader CH 0 (MHz)" -> [w417 w425]
      tunnel: "Fq Scan Endpoint (CH0)" -> [_ w424]
      tunnel: [w417 w423] -> w208
      tunnel: "Gain CH 0 (%)" -> [w416 w422]
      tunnel: "Gain Scan Endpoint (CH0)" -> [_ w421]
      tunnel: [w416 w420] -> w292
      tunnel: "Gain Scan Step Size % (CH0)" -> [_ w419]
      tunnel: w273 -> [_ w418]
      frame False {
        n130 = local write "write time ch0"(FALSE) -> ()
      }
      frame True {
        n131 = case shown="True" w418 {
          tunnel: w425 -> [w429 w443]
          tunnel: w424 -> [_ w441]
          tunnel: w426 -> [_ w442]
          tunnel: [w429 w440] -> w423
          tunnel: w422 -> [w428 w438]
          tunnel: w421 -> [_ w435]
          tunnel: w419 -> [_ w437]
          tunnel: [w428 w436] -> w420
          frame False {
            n132 = local write "write time ch0"(FALSE) -> ()
          }
          frame True {
            n133 = call "Ramp_to_setpoint_subvi.vi"("Numeric"=w437, "Scan to Fq (CH0)"=w435, "Wave Reader CH 0 (Y)"=w438) -> ("Array"=w436:dbl[])  [unwired: 8 in]
            n134 = call "Ramp_to_setpoint_subvi.vi"("Numeric"=w442, "Scan to Fq (CH0)"=w441, "Wave Reader CH 0 (Y)"=w443) -> ("Array"=w440:dbl[])  [unwired: 8 in]
            n135 = Equal?(x=w435, y=w436) -> (x = y?=w434:bool[])
            n136 = And Array Elements(Boolean array=w434) -> (logical AND=w431:bool)
            n137 = Equal?(x=w440, y=w441) -> (x = y?=w439:bool[])
            n138 = And Array Elements(Boolean array=w439) -> (logical AND=w432:bool)
            n139 = And(x=w432, y=w431) -> (x .and. y?=w433:bool)
            n140 = case shown="True" w433 {
              frame False {
              }
              frame True {
                n141 = local write "Scan CH0"(FALSE) -> ()
              }
            }
            n142 = local write "write time ch0"(TRUE) -> ()
          }
        }
      }
    }
    n143 = case shown="True" w271 {
      tunnel: w205 -> [_ w377]
      tunnel: "save path for power calibration (dialog if empty)" -> [_ w370]
      frame False {
      }
      frame True {
        n144 = Get Date/Time In Seconds() -> (seconds since 1Jan1904=w373:timestamp)
        n145 = To Double Precision Float(number=w373) -> (double precision float=w372:dbl)
        n146 = Index Array(array=w377, index=0) -> (element=w375:dbl)
        n147 = Format Date/Time String(time format string (%c)="%H:%M:%S%3u", seconds (now)=w373) -> (date/time string=w380:string)  [unwired: 1 in]
        n148 = Format Into String(format string="%#_10f", w375) -> (resulting string=w379:string)  [unwired: 2 in, 1 out]
        n149 = Format Into String(w372) -> (resulting string=w371:string)  [unwired: 3 in, 1 out]
        n150 = Build Array(w371, w380, w379) -> (w374:string[])
        n151 = call-poly <vilib>:"Write Delimited Spreadsheet.vi"("file path (dialog if empty)"=w370, "format (%s)"="%s" ("format (%.3f)"), "1D data"=w374, "append to file? (new file:F)"=TRUE, "delimiter (\\t)"="," ("delimiter (\\t)")) -> ()  [unwired: 9 in, 2 out]
      }
    }
    n152 = feedback-in #9("Gain CH 0 (%)") -> ()
    n153 = feedback #9() -> (w199:dbl[])  [unwired: 1 in]
    n154 = feedback #10() -> (w195:dbl[])  [unwired: 1 in]
    n155 = feedback-in #10("Gain CH 1 (%)") -> ()
    n156 = feedback #11() -> (w197:dbl[])  [unwired: 1 in]
    n157 = feedback-in #11("Wave Reader CH 1 (MHz)") -> ()
    n158 = feedback #12() -> (w200:dbl[])  [unwired: 1 in]
    n159 = feedback-in #12("Wave Reader CH 0 (MHz)") -> ()
    n160 = Not Equal?(x=w200, y="Wave Reader CH 0 (MHz)") -> (x != y?=w193:bool[])
    n161 = Not Equal?(x=w199, y="Gain CH 0 (%)") -> (x != y?=w192:bool[])
    n162 = Not Equal?(x=w197, y="Wave Reader CH 1 (MHz)") -> (x != y?=w191:bool[])
    n163 = Not Equal?(x=w195, y="Gain CH 1 (%)") -> (x != y?=w190:bool[])
    n164 = And(x="write time ch0", y="Record time for power sweep CH0") -> (x .and. y?=w267:bool)
    n165 = Multiply(x=1000000.0, y=w208) -> (x*y=w301:dbl[])
    n166 = local write "Wave Reader CH 1 (MHz)"(w205) -> ()
    n167 = local write "Gain CH 0 (%)"(w292) -> ()
    n168 = local write "Wave Reader CH 0 (MHz)"(w208) -> ()
    n169 = In Range and Coerce(upper limit=100.0, x=w292, lower limit=0.0) -> (coerced(x)=w295:dbl[])  [unwired: 1 out]
    n170 = Build Array(w193, w192, w191, w190) -> (w189:bool[][])
    n171 = In Range and Coerce(upper limit=100.0, x=w285, lower limit=0.0) -> (coerced(x)=w290:dbl[])  [unwired: 1 out]
    n172 = Divide(x=w295, y=100.0) -> (x/y=w258:dbl[])
    n173 = call "HF power flattener.vi"("CH 1 frequency"=w205, "CH 0 frequency"=w208) -> ("Normalized CH1"=w202:dbl[], "Normalized CH 0"=w206:dbl[])  [unwired: 2 in]
    n174 = local write "Gain CH 1 (%)"(w285) -> ()
    n175 = case shown="True" w267 {
      tunnel: w208 -> [_ w362]
      tunnel: "save path for power calibration (dialog if empty)" -> [_ w355]
      frame False {
      }
      frame True {
        n176 = Get Date/Time In Seconds() -> (seconds since 1Jan1904=w358:timestamp)
        n177 = To Double Precision Float(number=w358) -> (double precision float=w357:dbl)
        n178 = Index Array(array=w362, index=0) -> (element=w360:dbl)
        n179 = Format Date/Time String(time format string (%c)="%H:%M:%S%3u", seconds (now)=w358) -> (date/time string=w365:string)  [unwired: 1 in]
        n180 = Format Into String(format string="%#_10f", w360) -> (resulting string=w364:string)  [unwired: 2 in, 1 out]
        n181 = Format Into String(w357) -> (resulting string=w356:string)  [unwired: 3 in, 1 out]
        n182 = Build Array(w356, w365, w364) -> (w359:string[])
        n183 = call-poly <vilib>:"Write Delimited Spreadsheet.vi"("file path (dialog if empty)"=w355, "format (%s)"="%s" ("format (%.3f)"), "1D data"=w359, "append to file? (new file:F)"=TRUE, "delimiter (\\t)"="," ("delimiter (\\t)")) -> ()  [unwired: 9 in, 2 out]
      }
    }
    n184 = Multiply(x=1000000.0, y=w205) -> (x*y=w299:dbl[])
    n185 = case shown="False" "RF Power normalize" {
      tunnel: w258 -> [w325 w328]
      tunnel: [w325 w327] -> w207
      tunnel: w206 -> [_ w326]
      frame False {
      }
      frame True {
        n186 = Multiply(x=w328, y=w326) -> (x*y=w327:dbl[])
      }
    }
    n187 = Or Array Elements(Boolean array=w189) -> (logical OR=w188:bool)
    n188 = Divide(x=w290, y=100.0) -> (x/y=w203:dbl[])
    n189 = call "Power normalization.vi"("% of max CH 1"="% of max CH 1", "CH 1 frequency"=w205, "% of max CH 0"="% of max CH 0", "CH 0 frequency"=w208) -> ("Normalized CH1"=w253:dbl[], "Normalized CH 0"=w255:dbl[])
    n190 = Divide(x=w301, y=6104.0) -> (x/y=w264:fxp<+,20,13>[])
    n191 = Divide(x=w299, y=6104.0) -> (x/y=w263:fxp<+,20,13>[])
    n192 = Multiply(x=w207, y=w255) -> (x*y=w259:fxp<+,16,1>[])
    n193 = case shown="True" "RF Power normalize" {
      tunnel: [w321 w324] -> w204
      tunnel: w203 -> [w321 w323]
      tunnel: w202 -> [_ w322]
      frame False {
      }
      frame True {
        n194 = Multiply(x=w322, y=w323) -> (x*y=w324:dbl[])
      }
    }
    n195 = Multiply(x=w253, y=w204) -> (x*y=w254:fxp<+,16,1>[])
    n196 = case shown="True" w188 {
      selector: w188 -> [_ w335]
      tunnel: w312 -> [w333 w343]
      tunnel: w311 -> [w331 w342]
      tunnel: [w332 w341] -> w309
      tunnel: [w330 w340] -> w308
      tunnel: w264 -> [_ w339]
      tunnel: w263 -> [_ w338]
      tunnel: w259 -> [_ w337]
      tunnel: w254 -> [_ w336]
      tunnel: [w329 w334] -> w181
      frame False {
        n197 = xnode "Read/Write Control"("FPGA VI Reference In"=w333, "error in"=w331) -> ("FPGA VI Reference Out"=w332:refnum<k20>, "error out"=w330:errorcluster, "Update Params"=w329:bool)
      }
      frame True {
        n198 = xnode "Read/Write Control"("FPGA VI Reference In"=w343, "error in"=w342, "Update Params"=w335, "Wave 1 Set"=w339, "Amp 1 Set"=w337, "Wave 2 Set"=w338, "Amp 2"=w336) -> ("FPGA VI Reference Out"=w341:refnum<k20>, "error out"=w340:errorcluster, "Update Params"=w334:bool)
      }
    }
    "Boolean" <- w181
    n199 = In Range and Coerce(upper limit=u8 150, x="# of beams", lower limit=u8 1) -> (coerced(x)=w184:u8)  [unwired: 1 out]
    n200 = local write "# of beams"(w184) -> ()
    n201 = Multiply(x=u16 100, y="Time per beam in us") -> (x*y=w220:u16)
    n202 = Multiply(x=u16 100, y="Signal Delay (us)") -> (x*y=w217:u16)
    n203 = Subtract(x=w220, y="Remove transition edges") -> (x-y=w218:u16)
    n204 = Subtract(x=w218, y=w217) -> (x-y=w216:u16)
    n205 = xnode "Read/Write Control"("FPGA VI Reference In"=w309, "error in"=w308, "Size"=w184, "Timeshare"=w220, "Edge size"="Remove transition edges", "Pass selector"="Input pass through\nmode", "X Gains"="X Gains", "setpoint weighting"="setpoint weighting", "output range"="output range", "X reset? (F)"="X reset? (F)", "Signal Delay"=w217, "Data collection size"=w216) -> ("FPGA VI Reference Out"=w241:refnum<k20>, "error out"=w242:errorcluster)
    n206 = xnode "Read/Write Control"("FPGA VI Reference In"=w241, "error in"=w242, "Apply feedback"="Apply feedback", "Feedback scaling y"="Feedback scaling y", "Feedback scaling x"="Feedback scaling x", "Feedback scaling z"="Feedback scaling z", "Y Gains"="Y Gains", "setpoint weighting 2"="setpoint weighting 2", "output range 2"="output range 2", "Y reset? (F)"="Y reset? (F)", "Z Gains"="Z Gains", "setpoint weighting 3"="setpoint weighting 3", "output range 3"="output range 3", "Z reset? (F)"="Z reset? (F)", "Set Point Initialization"="Set Point Initialization") -> ("FPGA VI Reference Out"=w240:refnum<k20>, "error out"=w238:errorcluster, "actions 2"=→"actions 2":T9, "output 2"=→"output 2":sgl, "error 2"=→"error 2":sgl, "actions 3"=→"actions 3":T9, "output 3"=→"output 3":sgl, "error 3"=→"error 3":sgl, "actions"=→"actions":T9, "output"=→"output":sgl, "error"=→"error":sgl, "Feedback scaling x"=→"X DC Offset Check":fxp<+,25,4>)
    n207 = Or(x="stop", y=w238) -> (x .or. y?=w244:bool)
    n208 = in-place {
      in-place-border: [w469] -> w245
      in-place-border: w244 -> [w467]
      n209 = in-place-dvr #13(w315) -> (w470:bool, w468:errorcluster)
      n210 = Compound Arithmetic op=OR(w467, w470, w468) -> (w469:bool)
      n211 = in-place-dvr #13(w469) -> ()  [unwired: 2 out]
    }
    n212 = Wait (ms)(milliseconds to wait=u32 33) -> ()  [unwired: 1 out]
  }
  n213 = Merge Errors(w10, w9) -> (w11:errorcluster)
  n214 = xnode "Read/Write Control"("FPGA VI Reference In"=w17, "error in"=w11, "stream.request state 2"=3) -> ("FPGA VI Reference Out"=w14:refnum<k20>, "error out"=w16:errorcluster)
  n215 = xnode "Close FPGA VI Reference"("FPGA VI Reference In"=w14, "error in"=w16) -> ("error out"=w24:errorcluster)
  n216 = call <vilib>:"Simple Error Handler.vi"("error in (no error)"=w24) -> ("error out"=→"Error Out":errorcluster)  [unwired: 4 in, 4 out]
